vi "Finalize Validation.vi"(8 "error in":errorcluster, 10 "validation information":T1={"Missing Modules"=variant(cluster{"ID":string, "Path":string}[] []), "Module Connection Map"=variant, "Unused Modules"=variant(cluster{"ID":string, "Path":string}[] [])}, 11 "routing and faulting in":T2 format="%.0x") -> (0 "error out":errorcluster, 3 "routing and faulting out":T2 format="%.0x")   [LabVIEW 2020, in "Routing and Faulting Scripting.lvlib"]
uses:
  Routing and Faulting Scripting.lvlib
  <vilib>/NI VeriStand/Custom Device API/Custom Device Item Ref.ctl
  Validation Information.ctl
  <vilib>/NI VeriStand/Custom Device API/Custom Device API.lvlib
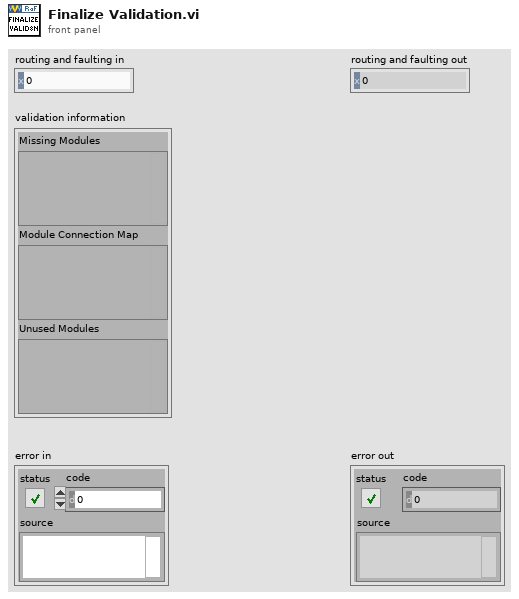
[diagram p1: front panel]
types:
  T1 = typedef "Routing and Faulting Scripting.lvlib/Validation Information.ctl" = cluster{"Missing Modules":variant, "Module Connection Map":variant, "Unused Modules":variant}
  T2 = typedef "Custom Device API.lvlib/Custom Device Item Ref.ctl" = u64
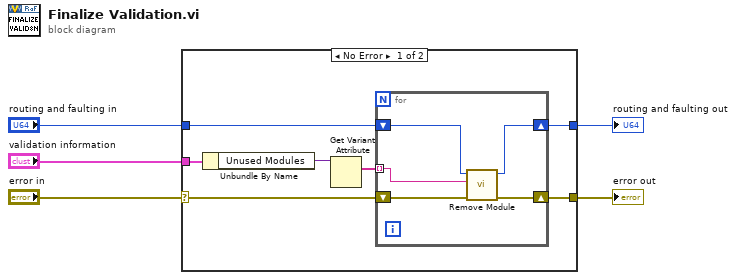
[diagram p0: block diagram]
diagram:
  n1 = case shown="No Error" "error in" {
    selector: "error in" -> [w12 w18]
    tunnel: "validation information" -> [w11 _]
    tunnel: "routing and faulting in" -> [w8 w19]
    tunnel: [w7 w18] -> w1
    tunnel: [w6 w19] -> w2
    frame No Error {
      n2 = Unbundle By Name(w11) -> ("Unused Modules"=w10:variant)
      n3 = Get Variant Attribute(Variant=w10) -> (names=w9:string[])  [unwired: 3 in, 3 out]
      n4 = for {
        tunnel: w9 -> [w16] mode=indexing
        shift-right: [w15] -> w6
        shift-left: w8 -> [w14]
        shift-right: [w13] -> w7
        shift-left: w12 -> [w17]
        n5 = call "Remove Module.vi"("error in"=w17, "module path"=w16, "routing and faulting in"=w14) -> ("error out"=w13:errorcluster, "routing and faulting out"=w15:T2)  [unwired: 7 in]
      }
    }
    frame Error {
    }
  }
  "routing and faulting out" <- w2
  "error out" <- w1
